vi "RESTful Control Direction To Text.vi"(1 "Indicator?":bool) -> (0 "Boolean Text":string)   [LabVIEW 2020]
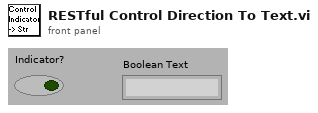
[diagram p1: front panel]
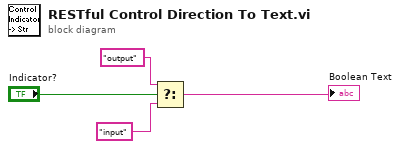
[diagram p0: block diagram]
diagram:
  n1 = Select(t="output", s="Indicator?", f="input") -> (s? t:f=→"Boolean Text":string)
